vi "Destroy.vi"(0 "reference in":refnum<class "Interface.lvclass">, 5 "error in (no error)":errorcluster) -> (14 "reference out":refnum<class "Interface.lvclass">, 19 "error out":errorcluster)   [LabVIEW 2013, in "Interface.lvclass"]
doc: "Destructor."
uses:
  Interface.lvclass
  <vilib>/addons/_AddQ/G#Interface/G#Interface.lvclass
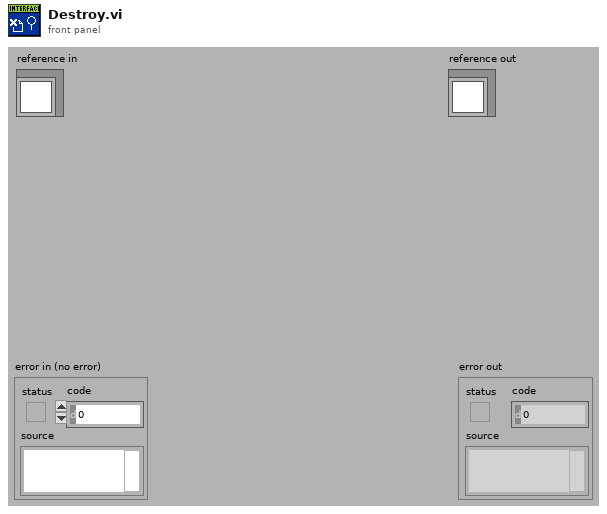
[diagram p1: front panel]
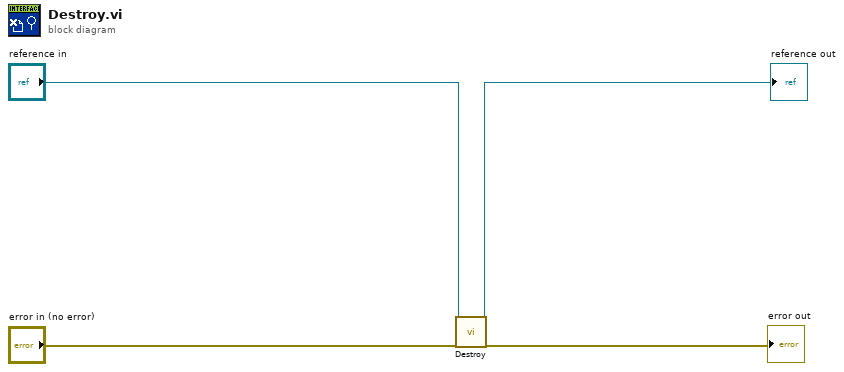
[diagram p0: block diagram]
diagram:
  n1 = call-parent "Destroy.vi"("reference in"="reference in", "error in (no error)"="error in (no error)") -> ("reference out"=→"reference out":refnum<class "Interface.lvclass">, "error out"=→"error out":errorcluster)  [unwired: 16 in]
